vi "CalculateSINHalfTheta.vi"(11 "cosHalfTheta":dbl) -> (0 "sinHalfTheta < 0.001":bool, 3 "sinHalfTheta":dbl)   [LabVIEW 2016]
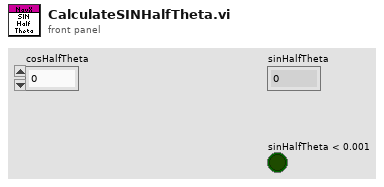
[diagram p1: front panel]
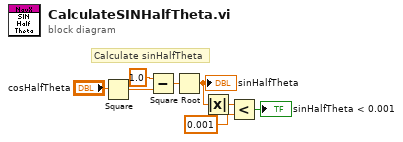
[diagram p0: block diagram]
diagram:
  # "Calculate sinHalfTheta"
  n1 = Square(x="cosHalfTheta") -> (x^2=w7:dbl)
  n2 = Subtract(x=1.0, y=w7) -> (x-y=w8:dbl)
  n3 = Square Root(x=w8) -> (sqrt(x)=w4:dbl)
  "sinHalfTheta" <- w4
  n4 = Absolute Value(x=w4) -> (abs(x)=w3:dbl)
  n5 = Less?(x=w3, y=0.001) -> (x < y?=→"sinHalfTheta < 0.001":bool)
